vi "setCalibration.vi"(8 "error in (no error)":errorcluster, 10 "calibration":cluster{"gradient":dbl, "offset":dbl}, 11 "Channel.lvclass in":refnum<class "Channel.lvclass">) -> (0 "error out":errorcluster, 3 "Channel.lvclass out":refnum<class "Channel.lvclass">)   [LabVIEW 2011, in "Tools.lvlib" / "DatabaseHelpers.lvlib" / "Channel.lvclass"]
uses:
  Channel.lvclass
  Channel.lvclass/Channel.ctl
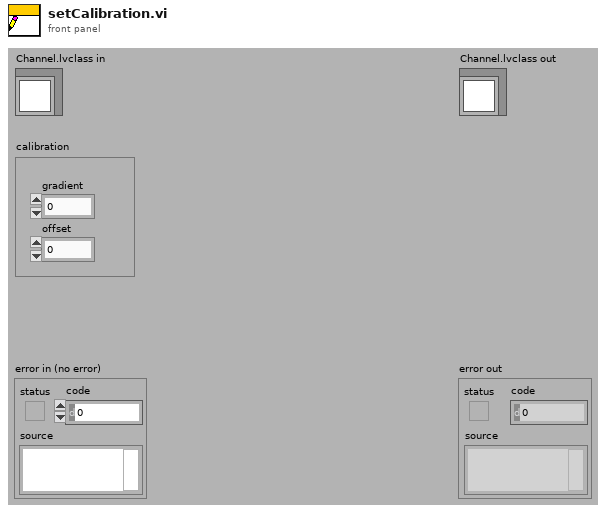
[diagram p1: front panel]
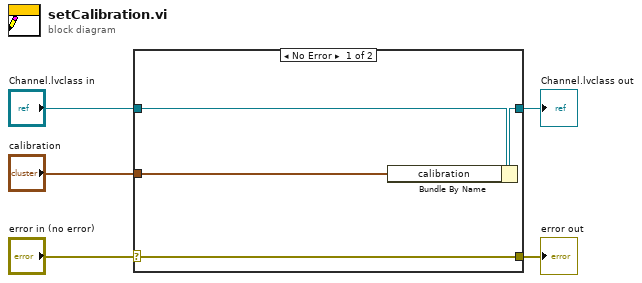
[diagram p0: block diagram]
diagram:
  n1 = case shown="No Error" "error in (no error)" {
    selector: "error in (no error)" -> [w9 w10]
    tunnel: [w9 w10] -> w4
    tunnel: [w7 w11] -> w2
    tunnel: "Channel.lvclass in" -> [w8 w11]
    tunnel: "calibration" -> [w6 _]
    frame No Error {
      n2 = Bundle By Name(cluster=w8, "calibration"=w6) -> (w7:refnum<class "Channel.lvclass">)
    }
    frame Error {
    }
  }
  "error out" <- w4
  "Channel.lvclass out" <- w2
